vi "Read TimeN.vi"(8 "error in (no error)":errorcluster, 11 "SquareBattle Arena in":refnum<class "SquareBattle Arena.lvclass">) -> (0 "error out":errorcluster, 2 "TimeN":refnum<notifier>, 3 "SquareBattle Arena out":refnum<class "SquareBattle Arena.lvclass">)   [LabVIEW 2014, in "SquareBattle Arena.lvlib" / "SquareBattle Arena.lvclass"]
uses:
  SquareBattle Arena.lvclass
  SquareBattle Arena.lvclass/SquareBattle Arena.ctl
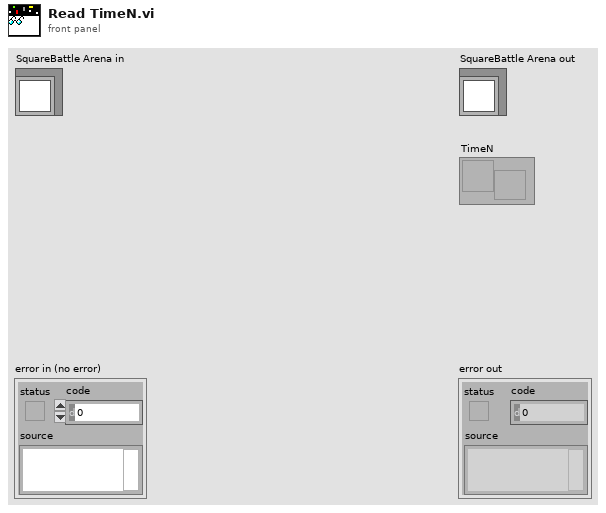
[diagram p1: front panel]
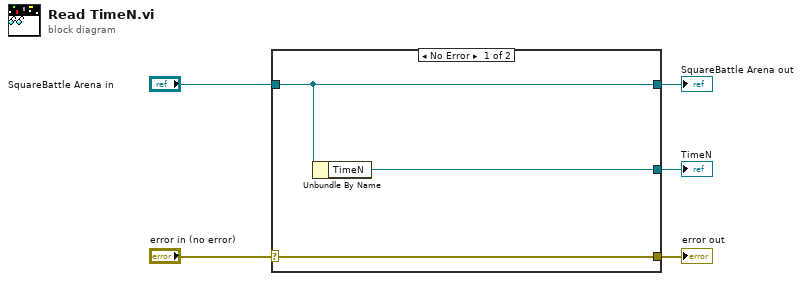
[diagram p0: block diagram]
diagram:
  n1 = case shown="No Error" "error in (no error)" {
    selector: "error in (no error)" -> [w8 w9]
    tunnel: [w8 w9] -> w4
    tunnel: [w7 w10] -> w2
    tunnel: "SquareBattle Arena in" -> [w7 w10]
    tunnel: [w6 _] -> w1
    frame No Error {
      n2 = Unbundle By Name(w7) -> ("TimeN"=w6:refnum<notifier>)
    }
    frame Error {
    }
  }
  "error out" <- w4
  "SquareBattle Arena out" <- w2
  "TimeN" <- w1
